vi "VI Folder Action Template.vi"(8 "error in (no error)":errorcluster, 11 "VI Folder":path) -> (0 "error out":errorcluster, 3 "VI List":path[](array[path]))   [LabVIEW 2014, in "SLL Application.lvlib"]
doc: "This VI can be used to find the list of broken VIs in a folder. This also returns VIs which are of higher LabVIEW version than the currently used LabVIEW version."
uses:
  SLL Application.lvlib
panel:
  out "Progress":i32
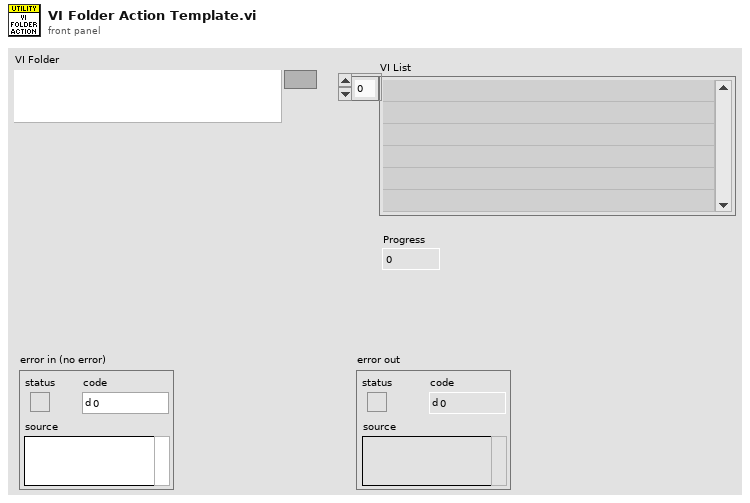
[diagram p1: front panel]
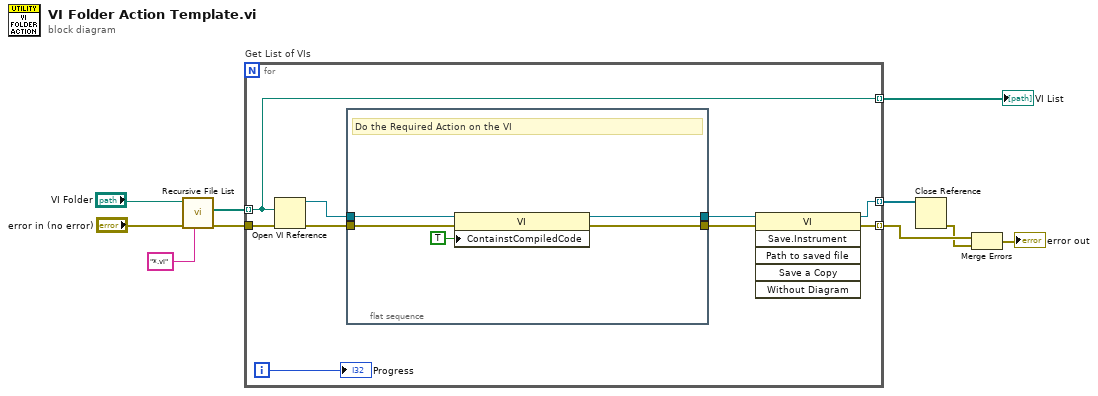
[diagram p0: block diagram]
diagram:
  n1 = call <vilib>:"Recursive File List.vi"("pattern"="*.vi", "error in (no error)"="error in (no error)", "Folder Path"="VI Folder") -> ("error out"=w4:errorcluster, "All Files in Dir"=w7:path[])  [unwired: 4 in, 3 out]
  n2 = for "Get List of VIs" {
    tunnel: [w11] -> w10 mode=indexing
    tunnel: w7 -> [w18] mode=indexing
    tunnel: [w18] -> w6 mode=indexing
    tunnel: w4 -> [w17]
    tunnel: [w13] -> w3 mode=indexing
    i -> [w14]
    n3 = Open VI Reference(vi path=w18, error in (no error)=w17) -> (vi reference=w19:refnum<vi>, error out=w16:errorcluster)  [unwired: 4 in]
    n4 = flat-sequence {
      tunnel: w19 -> [w24]
      tunnel: w16 -> [w23]
      tunnel: [w22] -> w15
      tunnel: [w21] -> w12
      frame #0 {
        # "Do the Required Action on the VI"
        n5 = property class="VI"(reference=w24, error in=w23, "ContainstCompiledCode"=TRUE ("Contains Compiled Code")) -> (reference out=w21:refnum<vi>, error out=w22:errorcluster)
      }
    }
    n6 = invoke class="VI" method="Save.Instrument"(reference=w12, error in=w15) -> (reference out=w11:refnum<vi>, error out=w13:errorcluster)  [unwired: 4 in, 4 out]
    "Progress" <- w14
  }
  "VI List" <- w6
  n7 = Close Reference(reference=w10) -> (error out=w2:errorcluster)  [unwired: 1 in]
  n8 = Merge Errors(w3, w2) -> (→"error out":errorcluster)
